vi "Mean Freq Curves.vi"(0 "Set of Freq samples":T1, 5 "Active Fit":bool) -> (14 "Mean Freq Curve":dbl[](array[numeric]), 15 "Max-Min error (Hz)":dbl, 16 "Max-Min error (% over Mean)":dbl, 17 "RMS of peak-peak value (Hz)":dbl format="%0.2f", 18 "RMS of peak-peak value (% over Mean)":dbl, 19 "StdDev%":dbl)   [LabVIEW 2014]
uses:
  <vilib>/Analysis/Matrix/Datatypes/RealMatrix.ctl
  <vilib>/Analysis/5stat.llb/RMS (DBL).vi
  <vilib>/imath/engines/lvmath2/RunTimeEngine/RangeToken/NIMS_Range.vi
  <instcachedir>/0/NIMS_Range_9BCE657718DF4976A877346C61F22738.lvgen/NIMS_Range_9BCE657718DF4976A877346C61F22738_001.vi
  <vilib>/imathl/engines/lvmath/Functions/Error Handling/Create Error.vi
  <vilib>/imath/engines/lvmath2/RunTimeEngine/BuiltInFunctions/polyfit/NIMS_[2o]_polyfit.vi
  <vilib>/imath/engines/lvmath2/RunTimeEngine/ErrorHandling/NIMS_Error From Error Code.vi
  <vilib>/imath/engines/lvmath2/RunTimeEngine/BuiltInFunctions/polyval/NIMS_polyval(GV,GM).vi
  <instcachedir>/0/NIMS_polyval(GV,GM)_E12556DC54744E0C81968744501C4F35.lvgen/NIMS_polyval(GV,GM)_E12556DC54744E0C81968744501C4F35_002.vi
  <vilib>/imath/engines/lvmath2/RunTimeEngine/NodeEndStatement/NIMS_NodeEndStatement_Output.vi
  <instcachedir>/0/NIMS_NodeEndStatement_Output_53EC0D466D134D7ABD903AC30B43404B.lvgen/NIMS_NodeEndStatement_Output_53EC0D466D134D7ABD903AC30B43404B_005.vi
  <vilib>/imath/engines/lvmath2/RunTimeEngine/ErrorHandling/NIMS_Finalize Error.vi
  <vilib>/Analysis/NI_AALBase.lvlib
  <vilib>/Analysis/NI_AALPro.lvlib
  <vilib>/Analysis/Matrix/NI_Matrix.lvlib
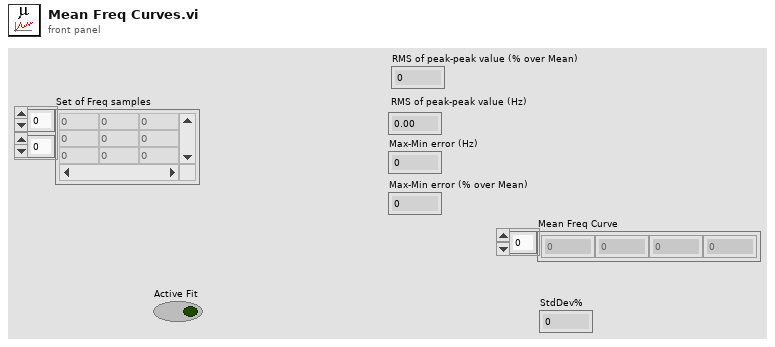
[diagram p1: front panel]
types:
  T1 = typedef "NI_Matrix.lvlib/RealMatrix.ctl" = dbl[][]
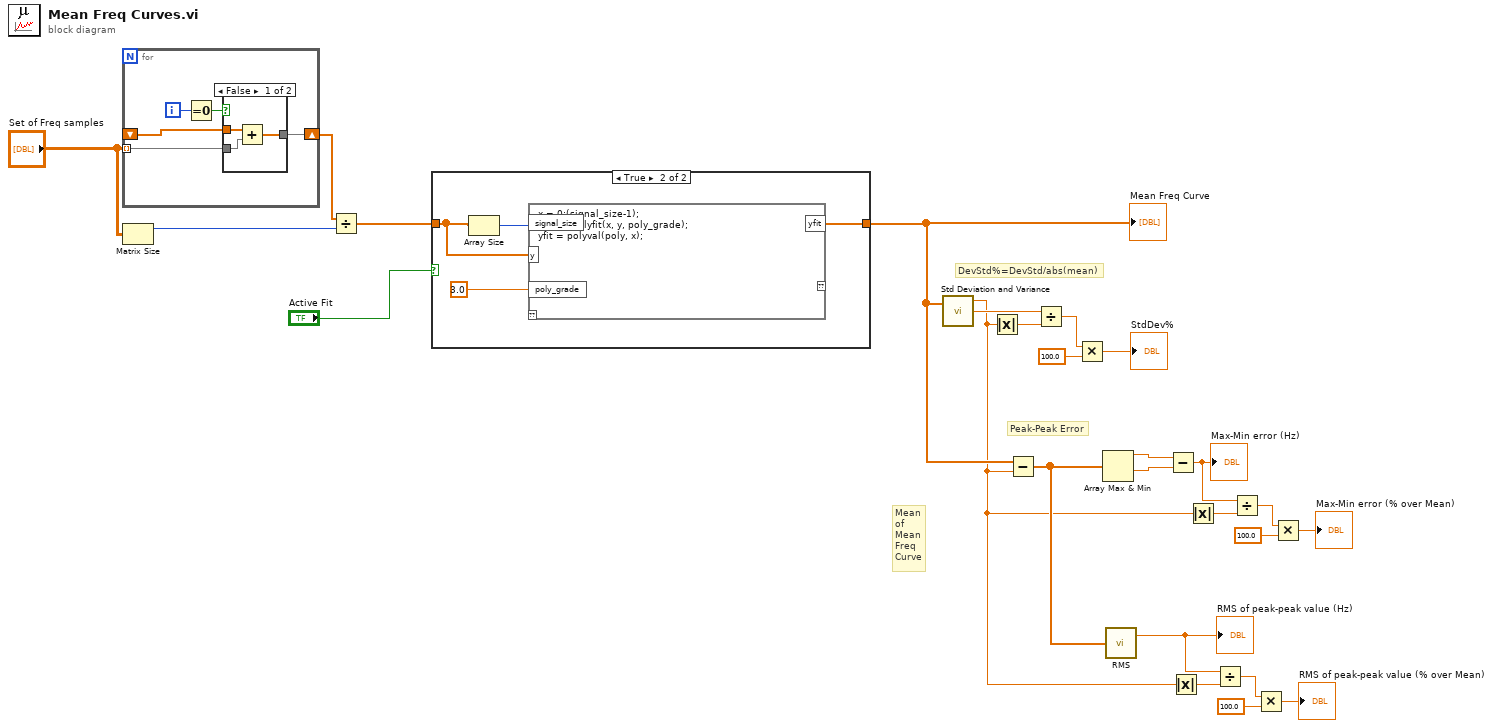
[diagram p0: block diagram]
diagram:
  # "Mean\nof \nMean\nFreq \nCurve"
  # "Peak-Peak Error"
  # "DevStd%=DevStd/abs(mean)"
  n1 = for {
    tunnel: "Set of Freq samples" -> [w27] mode=indexing
    shift-right: [w28] -> w24
    shift-left: _ -> [w26]
    i -> [w30]
    n2 = Equal To 0?(x=w30) -> (x = 0?=w29:bool)
    n3 = case shown="False" w29 {
      tunnel: [w31 w34] -> w28
      tunnel: w27 -> [w32 w34]
      tunnel: w26 -> [w33 _]
      frame False {
        n4 = Add(x=w33, y=w32) -> (x+y=w31:dbl[])
      }
      frame True {
      }
    }
  }
  n5 = Matrix Size(0:"Set of Freq samples") -> (1:w25:i32)  [unwired: 1 out]
  n6 = Divide(x=w24, y=w25) -> (x/y=w17:dbl[])
  n7 = case shown="True" "Active Fit" {
    tunnel: w17 -> [w35 w37]
    tunnel: [w35 w36] -> w15
    frame False {
    }
    frame True {
      n8 = Array Size(array=w37) -> (size(s)=w38:i32)
      n9 = mathscript code="x = 0:(signal_size-1);\npoly = polyfit(x, y, poly_grade); \nyfit = polyval(poly, x);"("signal_size"=w38, "y"=w37, "poly_grade"=3.0) -> ("yfit"=w36:dbl[])  [unwired: 1 in, 1 out]
    }
  }
  "Mean Freq Curve" <- w15
  n10 = call <vilib>:"Std Deviation and Variance.vi"("X"=w15) -> ("mean"=w1:dbl, "standard deviation"=w22:dbl)  [unwired: 1 in, 1 out]
  n11 = Absolute Value(x=w1) -> (abs(x)=w21:dbl)
  n12 = Subtract(x=w15, y=w1) -> (x-y=w14:dbl[])
  n13 = Divide(x=w22, y=w21) -> (x/y=w18:dbl)
  n14 = Multiply(x=w18, y=100.0) -> (x*y=→"StdDev%":dbl)
  n15 = Array Max & Min(array=w14) -> (max value=w13:dbl, min value=w12:dbl)  [unwired: 2 out]
  n16 = call-poly <vilib>:"RMS.vi"("X"=w14) -> ("rms value"=w2:dbl)  [unwired: 1 out]
  "RMS of peak-peak value (Hz)" <- w2
  n17 = Subtract(x=w13, y=w12) -> (x-y=w8:dbl)
  "Max-Min error (Hz)" <- w8
  n18 = Absolute Value(x=w1) -> (abs(x)=w6:dbl)
  n19 = Absolute Value(x=w1) -> (abs(x)=w11:dbl)
  n20 = Divide(x=w2, y=w6) -> (x/y=w4:dbl)
  n21 = Divide(x=w8, y=w11) -> (x/y=w9:dbl)
  n22 = Multiply(x=w4, y=100.0) -> (x*y=→"RMS of peak-peak value (% over Mean)":dbl)
  n23 = Multiply(x=w9, y=100.0) -> (x*y=→"Max-Min error (% over Mean)":dbl)
